vi "Method.vi"(4 "Value":refnum<class "Abs_U64 Integer.lvclass">) -> (1 "Result":refnum<class "Abs_Boolean.lvclass">)   [LabVIEW 2021, in "Not Equal 0_U64.lvclass"]
uses:
  Not Equal 0_U64.lvclass
  Abs_Types/U64 Integer/Abs_U64 Integer.lvclass
  Abs_Types/Boolean/Abs_Boolean.lvclass
  C:/TSA/LV_Abstract/Source/Functions/Support/Compare/One Term/U64/AbsComp_One Term_U64.lvclass
  C:/Program Files (x86)/National Instruments/LabVIEW 2021/vi.lib/TSA/Abstract Data Classes/Abs_Types/Boolean/Abs_Boolean.lvclass
  Support/Compare/One Term/U64/AbsComp_One Term_U64.lvclass/AbsComp_One Term_U64.ctl
  Support/Compare/One Term/U64/Properties/Write Numeric A.vi
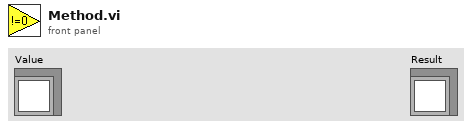
[diagram p1: front panel]
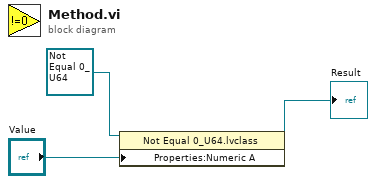
[diagram p0: block diagram]
diagram:
  n1 = property class="Not Equal 0_U64.lvclass"(reference=refnum<class "Not Equal 0_U64.lvclass"> refnum ("Greater 0_U64.lvclass"), "Properties:Numeric A"="Value") -> (reference out=→"Result":refnum<class "Not Equal 0_U64.lvclass">)  [unwired: 1 in, 1 out]
